vi "Performance Test.vi"() -> ()   [LabVIEW 2021]
uses:
  <vilib>/Platform/TimedLoop/XDataNode/wakeup.ctl
  <vilib>/Platform/TimedLoop/XDataNode/XDNodeRunTimeDep.lvlib
  <vilib>/Platform/TimedLoop/XDataNode/nitl_modes.ctl
  <vilib>/Platform/TimedLoop/XDataNode/timing_clust.ctl
  <vilib>/Platform/TimedLoop/XDataNode/XDataNode.xnode
  CIFChannels/Typedef/Direction.ctl
  CIFChannels/CIFChannels.lvclass
  ChannelCommon/typedef/FIFO Config.ctl
  ChannelCommon/ChannelCommon.lvlib
  ChannelCommon/typedef/TimeStamps.ctl
  CIF_NIChn_L2Enet.lvclass
  D:/dev/Packages/CIF_Channels_Core/src/CIF_NIChn/FIFO_U8_Multi/CIF_Fifo_U8_Multi.lvclass
  D:/dev/Packages/CIF_Channels_Core/src/CIF_NIChn/FIFO_U8/CIF_NIChn_Fifo_U8.lvclass
  D:/dev/Packages/CIF_Channels_Core/src/CIF_NIChn/NIChn/CIF_NIChn.lvclass
  D:/dev/Packages/CIF_Channels_Core/src/CIFChannels/CIFChannels.lvclass
  D:/dev/Packages/CIF_Channels_Core/src/CIF_NIChn/FIFO_L2Enet/CIF_NIChn_L2Enet.lvclass
  ChannelCommon/typedef/New FIFO Instance Configuration.ctl
  ChannelCommon/typedef/Benchmark Stats.ctl
panel:
  out "Timeout RW Inline":bool
  out "Write (us) 3":T1
  out "Flatten (us) 3":T1
  out "Read (us) 3":T1
  out "Unflatten (us) 3":T1
  out "pass":bool
  out "error out":errorcluster
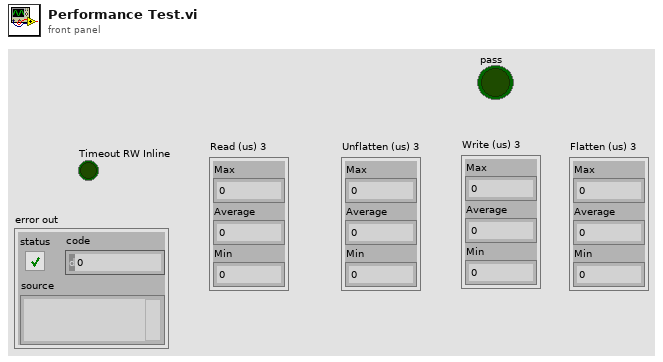
[diagram p1: front panel]
types:
  T1 = typedef "ChannelCommon.lvlib/Benchmark Stats.ctl" = cluster{"Max":i64, "Average":dbl, "Min":i64}
  T2 = typedef "ChannelCommon.lvlib/FIFO Config.ctl" = cluster{"Max Bytes/Msg":u64, "Max Msg/FIFO":u64, "Flags":u64}
  T3 = typedef "CIFChannels.lvclass/Direction.ctl" = enum16{"Publisher", "Subscriber"}
  T4 = typedef "ChannelCommon.lvlib/New FIFO Instance Configuration.ctl" = cluster{"Backpressure":bool, "Bytes/Message Override":u32, "Messages/FIFO Override":u32, "Custom Data":u8[]}
  T5 = typedef "ChannelCommon.lvlib/TimeStamps.ctl" = cluster{"ClockID":u8, "T0":i64, "T_Out":i64}
  T6 = typedef "XDNodeRunTimeDep.lvlib/timing_clust.ctl" = cluster{"Expected End [f-1]":u64, "Actual End [f-1]":u64, "Finished Late? [f-1]":bool, "Expected End [i-1]":u64, "Actual End [i-1]":u64, "Finished Late? [i-1]":bool, "Expected Start [i]":u64, "Actual Start [i]":u64, "Expected Start [f]":u64, "Actual Start [f]":u64, "Source Name":string, "Structure Name":string, "Period":i64, "Deadline":i64, "Offset":i64, "Start":i64, "Priority":i32, "Timeout":i32, "Mode":T7, "Wakeup Reason":T8, "Error":errorcluster, "Source Type":string, "Secondary Source Type":string, "Global End Time":u64, "Global Start Time":u64, "Frame Duration":u64, "Iteration Duration":u64, "Assigned CPU":i32, "I/O Scan Engine Mode":u32}
  T7 = typedef "XDNodeRunTimeDep.lvlib/nitl_modes.ctl" = enum32{"No Change", "Process missed periods, maintain original phase", "Discard missed periods, maintain original phase", "Process missed periods, ignore original phase", "Discard missed periods, ignore original phase"}
  T8 = typedef "XDNodeRunTimeDep.lvlib/wakeup.ctl" = enum32{"Normal", "Aborted", "Asynchronous wakeup", "Timing source error", "Timed loop error", "Timeout"}
  T9 = typedef "ChannelCommon.lvlib/New FIFO Instance Response.ctl" = cluster{"Publisher":string, "Custom Data":u8[]}
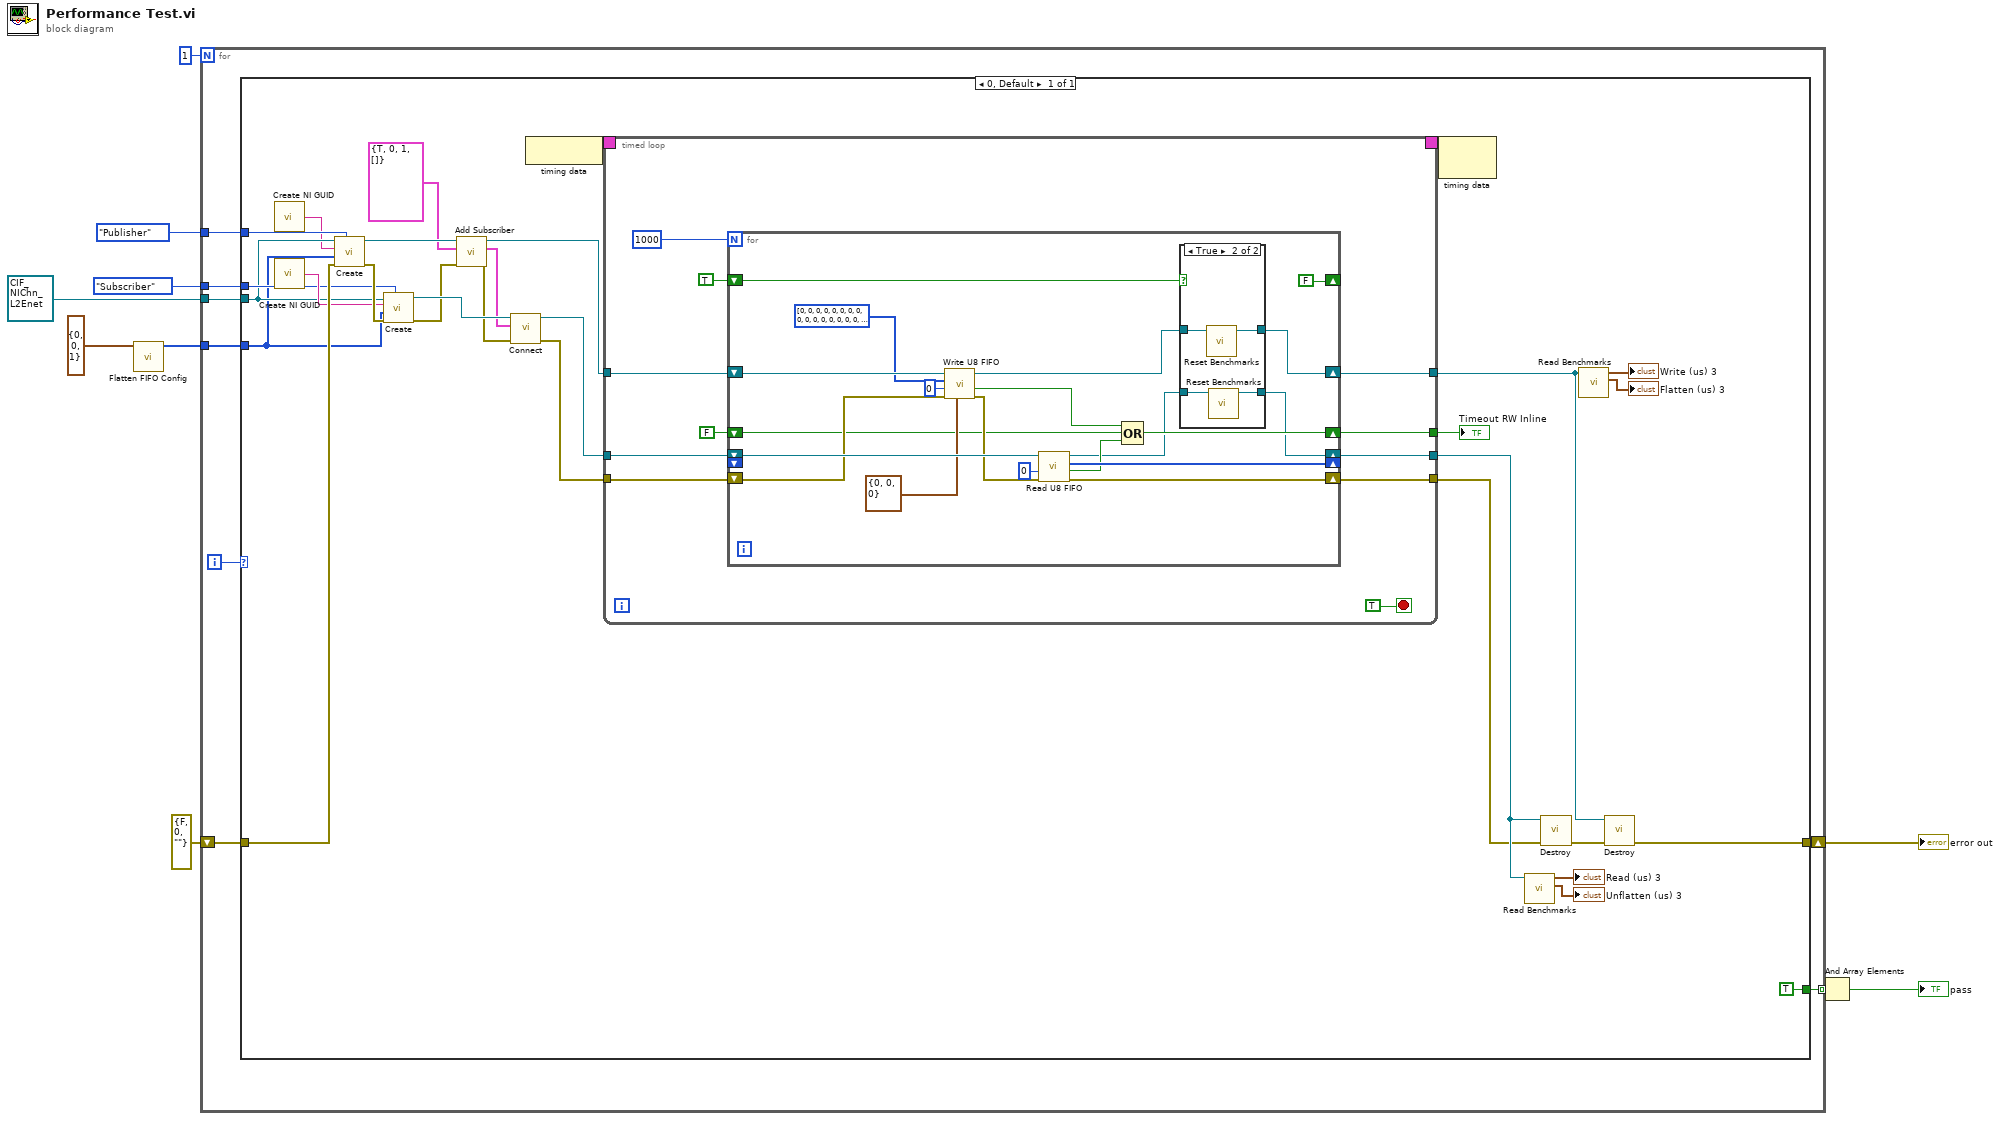
[diagram p0: block diagram]
diagram:
  n1 = call "Flatten FIFO Config.vi"("FIFO Config in"=T2 {"Max Bytes/Msg"=0, "Max Msg/FIFO"=0, "Flags"=1}) -> ("Flattened FIFO Config"=w2:u8[])  [unwired: 10 in]
  n2 = for {
    N: 1 -> [_]
    tunnel: [w18] -> w8 mode=indexing
    shift-right: [w17] -> w10
    shift-left: errorcluster {"status"=FALSE, "code"=0, "source"=""} ("error out") -> [w15]
    tunnel: Direction."Publisher" ("Direction") -> [w14]
    tunnel: Direction."Subscriber" ("Direction") -> [w13]
    tunnel: refnum<class "CIF_NIChn_L2Enet.lvclass"> refnum ("CIF_DAQ_DVR_Multi.lvclass") -> [w12]
    tunnel: w2 -> [w11]
    i -> [w16]
    n3 = case shown="0, Default" w16 {
      tunnel: [TRUE] -> w18
      tunnel: [w38] -> w17
      tunnel: w15 -> [w47]
      tunnel: w14 -> [w45]
      tunnel: w13 -> [w44]
      tunnel: w12 -> [w43]
      tunnel: w11 -> [w40]
      frame 0, Default {
        n4 = call <vilib>:"Create NI GUID.vi"() -> ("NI GUID"=w41:string)
        n5 = call <vilib>:"Create NI GUID.vi"() -> ("NI GUID"=w46:string)
        n6 = call-dynamic "Create.vi"("Direction"=w45, "error in (no error)"=w47, "Custom Config Data"=w40, "Name"=w41, "CIF_Fifo_U8 in"=w43) -> ("error out"=w48:errorcluster, "CIF_Fifo_U8 out"=w24:refnum<class "CIF_NIChn_L2Enet.lvclass">)  [unwired: 5 in]
        n7 = call-dynamic "Create.vi"("Direction"=w44, "error in (no error)"=w48, "Custom Config Data"=w40, "Name"=w46, "CIF_Fifo_U8 in"=w43) -> ("error out"=w21:errorcluster, "CIF_Fifo_U8 out"=w42:refnum<class "CIF_NIChn_L2Enet.lvclass">)  [unwired: 5 in]
        n8 = call-dynamic "Add Subscriber.vi"("error in (no error)"=w21, "New FIFO Instance Config"=T4 {"Backpressure"=TRUE, "Bytes/Message Override"=0, "Messages/FIFO Override"=1, "Custom Data"=[]}, "CIF_Fifo_U8 in"=w24) -> ("error out"=w20:errorcluster, "New FIFO Instance"=w22:T9, "CIF_Fifo_U8 out"=w23:refnum<class "CIF_NIChn_L2Enet.lvclass">)  [unwired: 6 in]
        n9 = call-dynamic "Connect.vi"("error in (no error)"=w20, "Connection"=w22, "CIFTag in"=w42) -> ("error out"=w32:errorcluster, "CIFTag out"=w33:refnum<class "CIF_NIChn_L2Enet.lvclass">)  [unwired: 7 in]
        n10 = node-c288() -> (w35:T6)
        n11 = timed-loop {
          timing: w35 -> [_]
          timing-out: [_] -> w34
          tunnel: w33 -> [w59]
          tunnel: w32 -> [w58]
          tunnel: [w56] -> w31
          tunnel: [w55] -> w30
          tunnel: [w50] -> w25
          tunnel: w23 -> [w53]
          tunnel: [w52] -> w27
          stop <- TRUE stop-if-true
          n12 = for {
            N: 1000 -> [_]
            shift-right: [w61] -> w56
            shift-left: w59 -> [w79]
            shift-right: [w78] -> w55
            shift-left: w58 -> [w75]
            shift-right: [w77] -> _
            shift-left: _ -> [_]
            shift-right: [w60] -> w52
            shift-left: w53 -> [w73]
            shift-right: [w68] -> w50
            shift-left: FALSE -> [w69]
            shift-right: [FALSE] -> _
            shift-left: TRUE -> [w65]
            n13 = call-dynamic "Write U8 FIFO.vi"("FIFO Timestamps"=T5 {"ClockID"=0, "T0"=0, "T_Out"=0}, "error in (no error)"=w75, "Timeout (ms)"=0, "Data in"=u8[] [0, 0, 0, 0, 0, 0, 0, 0, 0, 0, 0, 0, 0, 0, 0, 0, 0, 0, 0, 0, 0, 0, 0, 0, 0, 0, 0, 0, 0, 0, 0, 0, 0, 0, 0, 0, 0, 0, 0, 0, 0, 0, 0, 0, 0, 0, 0, 0, 0, 0, 0, 0, 0, 0, 0, 0, 0, 0, 0, 0, 0, 0, 0, 0, 0, 0, 0, 0, 0, 0, 0, 0, 0, 0, 0, 0, 0, 0, 0, 0, 0, 0, 0, 0, 0, 0, 0, 0, 0, 0, 0, 0, 0, 0, 0, 0, 0, 0, 0, 0, 0, 0, 0, 0, 0, 0, 0, 0, 0, 0, 0, 0, 0, 0, 0, 0, 0, 0, 0, 0, 0, 0, 0, 0, 0, 0, 0, 0, 0, 0, 0, 0, 0, 0, 0, 0, 0, 0, 0, 0, 0, 0, 0, 0, 0, 0, 0, 0, 0, 0, 0, 0, 0, 0, 0, 0, 0, 0, 0, 0, 0, 0, 0, 0, 0, 0, 0, 0, 0, 0, 0, 0, 0, 0, 0, 0, 0, 0, 0, 0, 0, 0, 0, 0, 0, 0, 0, 0, 0, 0, 0, 0, 0, 0, 0, 0, 0, 0, 0, 0, 0, 0, 0, 0, 0, 0, 0, 0, 0, 0, 0, 0, 0, 0, 0, 0, 0, 0, 0, 0, 0, 0, 0, 0, 0, 0, 0, 0, 0, 0, 0, 0, 0, 0, 0, 0, 0, 0, 0, 0, 0, 0, 0, 0, 0, 0, 0, 0, 0, 0, 0, 0, 0, 0, 0, 0, 0, 0, 0, 0, 0, 0, 0, 0, 0, 0, 0, 0, 0, 0, 0, 0, 0, 0, 0, 0, 0, 0, 0, 0, 0, 0, 0, 0, 0, 0, 0, 0, 0, 0, 0, 0, 0, 0, 0, 0, 0, 0, 0, 0, 0, 0, 0, 0, 0, 0, 0, 0, 0, 0, 0, 0, 0, 0, 0, 0, 0, 0, 0, 0, 0, 0, 0, 0, 0, 0, 0, 0, 0, 0, 0, 0, 0, 0, 0, 0, 0, 0, 0, 0, 0, 0, 0, 0, 0, 0, 0, 0, 0, 0, 0, 0, 0, 0, 0, 0, 0, 0, 0, 0, 0, 0, 0, 0, 0, 0, 0, 0, 0, 0, 0, 0, 0, 0, 0, 0, 0, 0, 0, 0, 0, 0, 0, 0, 0, 0, 0, 0, 0, 0, 0, 0, 0, 0, 0, 0, 0, 0, 0, 0, 0, 0, 0, 0, 0, 0, 0, 0, 0, 0, 0, 0, 0, 0, 0, 0, 0, 0, 0, 0, 0, 0, 0, 0, 0, 0, 0, 0, 0, 0, 0, 0, 0, 0, 0, 0, 0, 0, 0, 0, 0, 0, 0, 0, 0, 0, 0, 0, 0, 0, 0, 0, 0, 0, 0, 0, 0, 0, 0, 0, 0, 0, 0, 0, 0, 0, 0, 0, 0, 0, 0, 0, 0, 0, 0, 0, 0, 0, 0, 0, 0, 0, 0, 0, 0, 0, 0, 0, 0, 0, 0, 0, 0, 0, 0, 0, 0, 0, 0, 0, 0, 0, 0, 0, 0, 0, 0, 0, 0, 0, 0, 0, 0, 0, 0, 0, 0, 0, 0, 0, 0, 0, 0, 0, 0, 0, 0, 0, 0, 0, 0, 0, 0, 0, 0, 0, 0, 0, 0, 0, 0, 0, 0, 0, 0, 0, 0, 0, 0, 0, 0, 0, 0, 0, 0, 0, 0, 0, 0, 0, 0, 0, 0, 0, 0, 0, 0, 0, 0, 0, 0, 0, 0, 0, 0, 0, 0, 0, 0, 0, 0, 0, 0, 0, 0, 0, 0, 0, 0, 0, 0, 0, 0, 0, 0, 0, 0, 0, 0, 0, 0, 0, 0, 0, 0, 0, 0, 0, 0, 0, 0, 0, 0, 0, 0, 0, 0, 0, 0, 0, 0, 0, 0, 0, 0, 0, 0, 0, 0, 0, 0, 0, 0, 0, 0, 0, 0, 0, 0, 0, 0, 0, 0, 0, 0, 0, 0, 0, 0, 0, 0, 0, 0, 0, 0, 0, 0, 0, 0, 0, 0, 0, 0, 0, 0, 0, 0, 0, 0, 0, 0, 0, 0, 0, 0, 0, 0, 0, 0, 0, 0, 0, 0, 0, 0, 0, 0, 0, 0, 0, 0, 0, 0, 0, 0, 0, 0, 0, 0, 0, 0, 0, 0, 0, 0, 0, 0, 0, 0, 0, 0, 0, 0, 0, 0, 0, 0, 0, 0, 0, 0, 0, 0, 0, 0, 0, 0, 0, 0, 0, 0, 0, 0, 0, 0, 0, 0, 0, 0, 0, 0, 0, 0, 0, 0, 0, 0, 0, 0, 0, 0, 0, 0, 0, 0, 0, 0, 0, 0, 0, 0, 0, 0, 0, 0, 0, 0, 0, 0, 0, 0, 0, 0, 0, 0, 0, 0, 0, 0, 0, 0, 0, 0, 0, 0, 0, 0, 0, 0, 0, 0, 0, 0, 0, 0, 0, 0, 0, 0, 0, 0, 0, 0, 0, 0, 0, 0, 0, 0, 0, 0, 0, 0, 0, 0, 0, 0, 0, 0, 0, 0, 0, 0, 0, 0, 0, 0, 0, 0, 0, 0, 0, 0, 0, 0, 0, 0, 0, 0, 0, 0, 0, 0, 0, 0, 0, 0, 0, 0, 0, 0, 0, 0, 0, 0, 0, 0, 0, 0, 0, 0, 0, 0, 0, 0, 0, 0, 0, 0, 0, 0, 0, 0, 0, 0, 0, 0, 0, 0, 0, 0, 0, 0, 0, 0, 0, 0, 0, 0, 0, 0, 0, 0, 0, 0, 0, 0, 0, 0, 0, 0, 0, 0, 0, 0, 0, 0, 0, 0, 0, 0, 0, 0, 0, 0, 0, 0, 0, 0, 0, 0, 0, 0, 0, 0, 0, 0, 0, 0, 0, 0, 0, 0, 0, 0, 0, 0, 0, 0, 0, 0, 0, 0, 0, 0, 0, 0, 0, 0, 0, 0, 0, 0, 0, 0, 0, 0, 0, 0, 0, 0, 0, 0, 0, 0, 0, 0, 0, 0, 0, 0, 0, 0, 0, 0, 0, 0, 0, 0, 0, 0, 0, 0, 0, 0, 0, 0, 0, 0, 0, 0, 0, 0, 0, 0, 0, 0, 0, 0, 0, 0, 0, 0, 0, 0, 0, 0, 0, 0, 0, 0, 0, 0, 0, 0, 0, 0, 0, 0, 0, 0, 0, 0, 0, 0, 0, 0, 0, 0, 0, 0, 0, 0, 0, 0, 0, 0, 0, 0, 0, 0, 0, 0, 0, 0, 0, 0, 0, 0, 0, 0, 0, 0, 0, 0, 0, 0, 0, 0, 0, 0, 0, 0, 0, 0, 0, 0, 0, 0, 0, 0, 0, 0, 0, 0, 0, 0, 0, 0, 0, 0, 0, 0, 0, 0, 0, 0, 0, 0, 0, 0, 0, 0, 0, 0, 0, 0, 0, 0, 0, 0, 0, 0, 0, 0, 0, 0, 0, 0, 0, 0, 0, 0, 0, 0, 0, 0, 0, 0, 0, 0, 0, 0, 0, 0, 0, 0, 0, 0, 0, 0, 0, 0, 0, 0, 0, 0, 0, 0, 0, 0, 0, 0, 0, 0, 0, 0, 0, 0, 0, 0, 0, 0, 0, 0, 0, 0, 0, 0, 0, 0, 0, 0, 0, 0, 0, 0, 0, 0, 0, 0, 0, 0, 0, 0, 0, 0, 0, 0, 0, 0, 0, 0, 0, 0, 0, 0, 0, 0, 0, 0, 0, 0, 0, 0, 0, 0, 0, 0, 0, 0], "CIF_Fifo_U8 in"=w73) -> ("error out"=w74:errorcluster, "timed out?"=w67:bool, "CIF_Fifo_U8 out"=w63:refnum<class "CIF_NIChn_L2Enet.lvclass">)  [unwired: 3 in, 1 out]
            n14 = call-dynamic "Read U8 FIFO.vi"("error in (no error)"=w74, "Timeout (ms)"=0, "CIFFIFO in"=w79) -> ("error out"=w78:errorcluster, "timed out?"=w70:bool, "Data out"=w77:u8[], "CIFFIFO out"=w62:refnum<class "CIF_NIChn_L2Enet.lvclass">)  [unwired: 4 in, 1 out]
            n15 = Compound Arithmetic op=OR(w67, w69, w70) -> (w68:bool)
            n16 = case shown="True" w65 {
              tunnel: w63 -> [w81 w85]
              tunnel: [w81 w84] -> w60
              tunnel: w62 -> [w80 w83]
              tunnel: [w80 w82] -> w61
              frame False {
              }
              frame True {
                n17 = call "Reset Benchmarks.vi"("CIFChannels in"=w85) -> ("CIFChannels out"=w84:refnum<class "CIF_NIChn_L2Enet.lvclass">)  [unwired: 9 in, 1 out]
                n18 = call "Reset Benchmarks.vi"("CIFChannels in"=w83) -> ("CIFChannels out"=w82:refnum<class "CIF_NIChn_L2Enet.lvclass">)  [unwired: 9 in, 1 out]
              }
            }
          }
        }
        "Timeout RW Inline" <- w25
        n19 = node-c288(w34) -> ()  [unwired: 1 out]
        n20 = call "Read Benchmarks.vi"("CIFChannels in"=w31) -> ("Flatten (us)"=→"Unflatten (us) 3":T1, "Channel R/W (us)"=→"Read (us) 3":T1)  [unwired: 9 in]
        n21 = call-dynamic "Destroy.vi"("error in (no error)"=w30, "CIF_Fifo_U8 in"=w31) -> ("error out"=w39:errorcluster)  [unwired: 8 in, 1 out]
        n22 = call "Read Benchmarks.vi"("CIFChannels in"=w27) -> ("Flatten (us)"=→"Flatten (us) 3":T1, "Channel R/W (us)"=→"Write (us) 3":T1)  [unwired: 9 in]
        n23 = call-dynamic "Destroy.vi"("error in (no error)"=w39, "CIF_Fifo_U8 in"=w27) -> ("error out"=w38:errorcluster)  [unwired: 8 in, 1 out]
      }
    }
  }
  "error out" <- w10
  n24 = And Array Elements(Boolean array=w8) -> (logical AND=→"pass":bool)
